vi "runXY.vi"   [LabVIEW 2013]
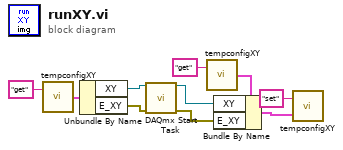
[diagram p0: block diagram]
diagram:
  n1 = call "tempconfigXY.vi"("command"="get") -> ("Temp Config out"=w4:cluster{" XY":refnum<k21>, "E_XY":errorcluster})  [unwired: 1 in]
  n2 = Unbundle By Name(w4) -> ("XY"=w5:refnum<k21>, "E_XY"=w6:errorcluster)
  n3 = call <vilib>:"DAQmx Start Task.vi"("task/channels in"=w5, "error in"=w6) -> ("task out"=w8:refnum<k21>, "error out"=w9:errorcluster)  [unwired: 12 in]
  n4 = call "tempconfigXY.vi"("command"="get") -> ("Temp Config out"=w7:cluster{" XY":refnum<k21>, "E_XY":errorcluster})  [unwired: 1 in]
  n5 = Bundle By Name(cluster=w7, "XY"=w8, "E_XY"=w9) -> (w10:cluster{" XY":refnum<k21>, "E_XY":errorcluster})
  n6 = call "tempconfigXY.vi"("Temp Config in"=w10, "command"="set") -> ()  [unwired: 1 out]
